vi "LVIS_GetTime.vi"(8 "Error In":errorcluster) -> (0 "Error out":errorcluster, 3 "DateTime":string)   [LabVIEW 2015]
doc: "Aquires the current Date/Time from the Data Commander if avaliable, else uses local PC time."
uses:
  Globals/LVIS_DcGlobals.vi
  Globals/LVIS_IsGlobal.vi
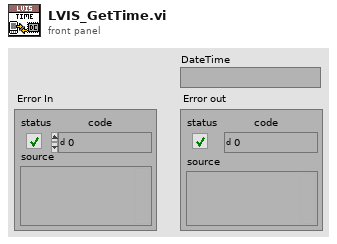
[diagram p1: front panel]
types:
  T1 = enum16{"Standard", "Buffered", "CRLF", "Immediate"}
  T2 = typedef "LVIS_SAF Status.ctl" = u16
  T3 = cluster{"ConnTimeout":string, "TxTimeout":string, "RxTimeout":string, "Port":string, "Map":string}
  T4 = cluster{"DCIP":string, "BackupFile":string, "ErrorLog":string, "FilePosition":string}
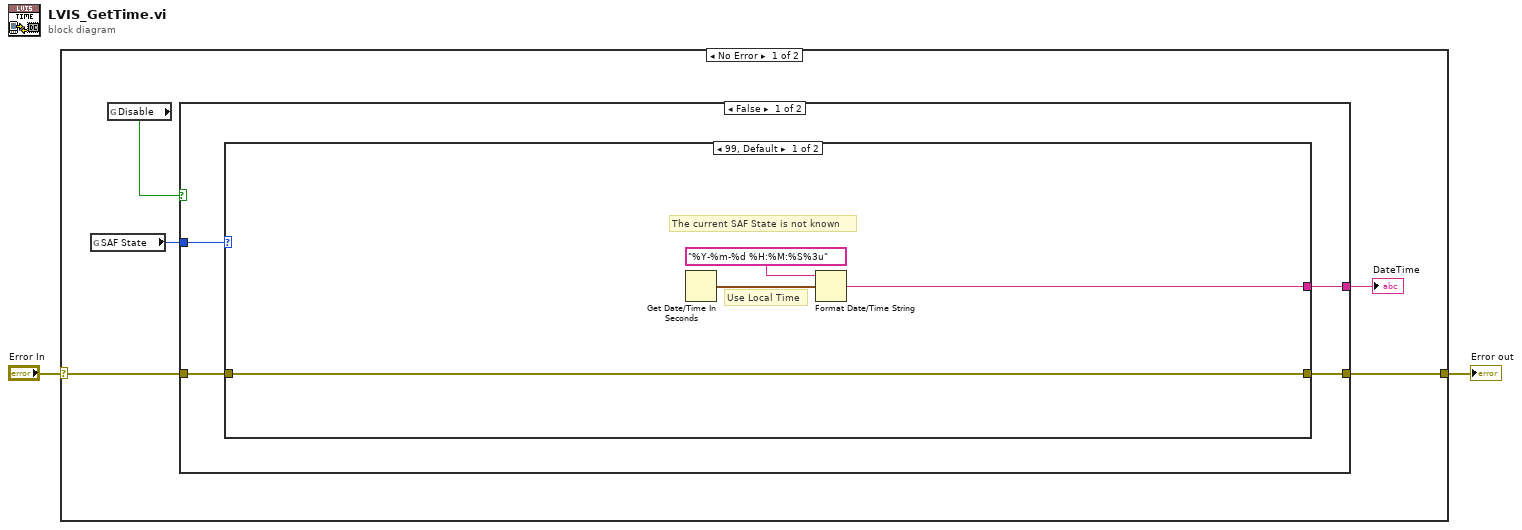
[diagram p0: block diagram]
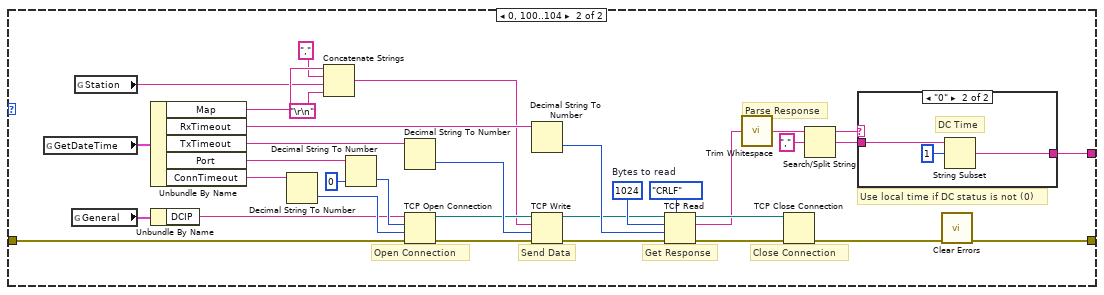
[diagram p2: hidden frame]
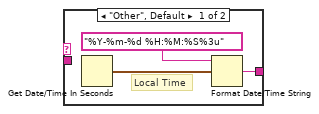
[diagram p3: hidden frame]
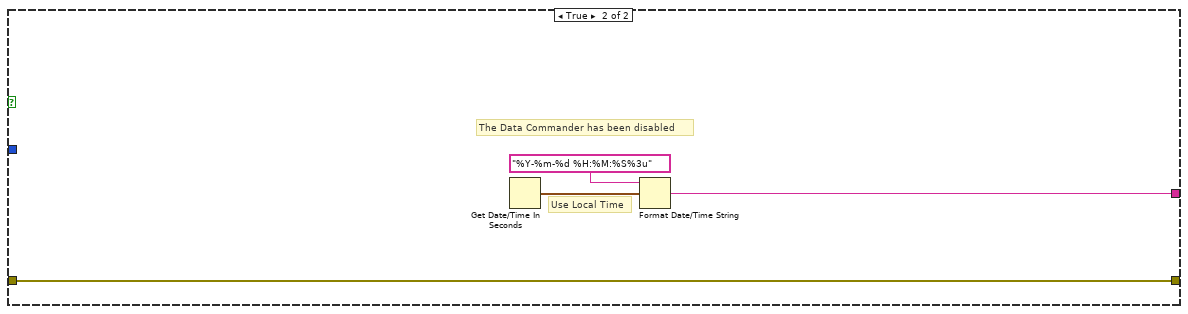
[diagram p4: hidden frame]
diagram:
  n1 = case shown="No Error" "Error In" {
    selector: "Error In" -> [w7 w60]
    tunnel: [w5 w60] -> w1
    frame No Error {
      n2 = global read "LVIS_DcGlobals.vi" "SAF State"() -> (w3:T2)
      n3 = global read "LVIS_DcGlobals.vi" "Disable"() -> (w4:bool)
      n4 = case shown="False" w4 {
        tunnel: w7 -> [w9 w56]
        tunnel: [w11 w57] -> w6
        tunnel: [w10 w56] -> w5
        tunnel: w3 -> [w8 _]
        frame False {
          n5 = case shown="99, Default" w8 {
            tunnel: [w12 w49] -> w11
            tunnel: [w15 w48] -> w10
            tunnel: w9 -> [w15 w17]
            frame 99, Default {
              # "The current SAF State is not known"
              # "Use Local Time"
              n6 = Get Date/Time In Seconds() -> (seconds since 1Jan1904=w14:timestamp)
              n7 = Format Date/Time String(time format string (%c)="%Y-%m-%d %H:%M:%S%3u", seconds (now)=w14) -> (date/time string=w12:string)  [unwired: 1 in]
            }
            frame 0, 100..104 {
              w33 = 1024  # Bytes to read
              # "Use local time if DC status is not (0)"
              # "Close Connection"
              # "Get Response"
              # "Send Data"
              # "Open Connection"
              # "Parse Response"
              n8 = global read "LVIS_DcGlobals.vi" "GetDateTime"() -> (w34:T3)
              n9 = global read "LVIS_DcGlobals.vi" "General"() -> (w35:T4)
              n10 = global read "LVIS_IsGlobal.vi" "Station"() -> (w18:string)
              n11 = Unbundle By Name(w34) -> ("Map"=w23:string, "RxTimeout"=w26:string, "TxTimeout"=w42:string, "Port"=w37:string, "ConnTimeout"=w38:string)
              n12 = Unbundle By Name(w35) -> ("DCIP"=w36:string)
              n13 = Decimal String To Number(string=w38) -> (number=w39:i32)  [unwired: 2 in, 1 out]
              n14 = Concatenate Strings(w23, "," ("string"), w18, "\r\n") -> (w21:string)
              n15 = Decimal String To Number(string=w37, default (0L)=u16 0 ("remote port or service name")) -> (number=w41:u16)  [unwired: 1 in, 1 out]
              n16 = Decimal String To Number(string=w42) -> (number=w43:i32)  [unwired: 2 in, 1 out]
              n17 = TCP Open Connection(address=w36, remote port or service name=w41, timeout ms (60000)=w39, error in (no error)=w17) -> (connection ID=w30:refnum<k5>, error out=w31:errorcluster)  [unwired: 1 in]
              n18 = Decimal String To Number(string=w26) -> (number=w44:i32)  [unwired: 2 in, 1 out]
              n19 = TCP Write(connection ID=w30, data in=w21, error in (no error)=w31, 9:w43) -> (connection ID out=w29:refnum<k5>, error out=w25:errorcluster)  [unwired: 1 out]
              n20 = TCP Read(connection ID=w29, bytes to read=w33, error in (no error)=w25, 7:T1."CRLF" ("mode (standard)"), 9:w44) -> (connection ID out=w27:refnum<k5>, data out=w20:string, error out=w28:errorcluster)
              n21 = call <vilib>:"Trim Whitespace.vi"("string"=w20) -> ("trimmed string"=w45:string)  [unwired: 1 in]
              n22 = TCP Close Connection(connection ID=w27, error in (no error)=w28) -> (error out=w24:errorcluster)  [unwired: 1 in, 1 out]
              n23 = Search/Split String(string=w45, search string/char (-)=",") -> (substring before match=w19:string, match + rest of string=w46:string)  [unwired: 1 in, 1 out]
              n24 = case shown="\"0\"" w19 {
                tunnel: w46 -> [_ w55]
                tunnel: [w50 w53] -> w49
                frame "Other", Default {
                  # "Local Time"
                  n25 = Get Date/Time In Seconds() -> (seconds since 1Jan1904=w52:timestamp)
                  n26 = Format Date/Time String(time format string (%c)="%Y-%m-%d %H:%M:%S%3u", seconds (now)=w52) -> (date/time string=w50:string)  [unwired: 1 in]
                }
                frame "0" {
                  # "DC Time"
                  n27 = String Subset(string=w55, offset (0)=1) -> (substring=w53:string)  [unwired: 1 in]
                }
              }
              n28 = call <vilib>:"Clear Errors.vi"("error in (no error)"=w24) -> ("error out"=w48:errorcluster)  [unwired: 5 in, 1 out]
            }
          }
        }
        frame True {
          # "The Data Commander has been disabled"
          # "Use Local Time"
          n29 = Get Date/Time In Seconds() -> (seconds since 1Jan1904=w59:timestamp)
          n30 = Format Date/Time String(time format string (%c)="%Y-%m-%d %H:%M:%S%3u", seconds (now)=w59) -> (date/time string=w57:string)  [unwired: 1 in]
        }
      }
      "DateTime" <- w6
    }
    frame Error {
    }
  }
  "Error out" <- w1
